vi "Update Digital Acq. Parameters.vi"(8 "error in":errorcluster, 10 "Digital Acquisition Parameters":T1 {"Execution Task Frequency" scale=1.0..100.0}) -> (0 "error out":errorcluster)   [LabVIEW 2020]
doc: "Request to update the Acquisition module with the information required to acquire digital info.\n_____\nCreated using Delacor QMH Event Scripter 6.0.0.121."
uses:
  Shared/DigitalAcquisitionParameters__typedef.ctl
  Shared/Configuration for Acquisitions.lvlib
  Update Digital Acq. Parameters Argument--cluster.ctl
  Acquisition.lvlib
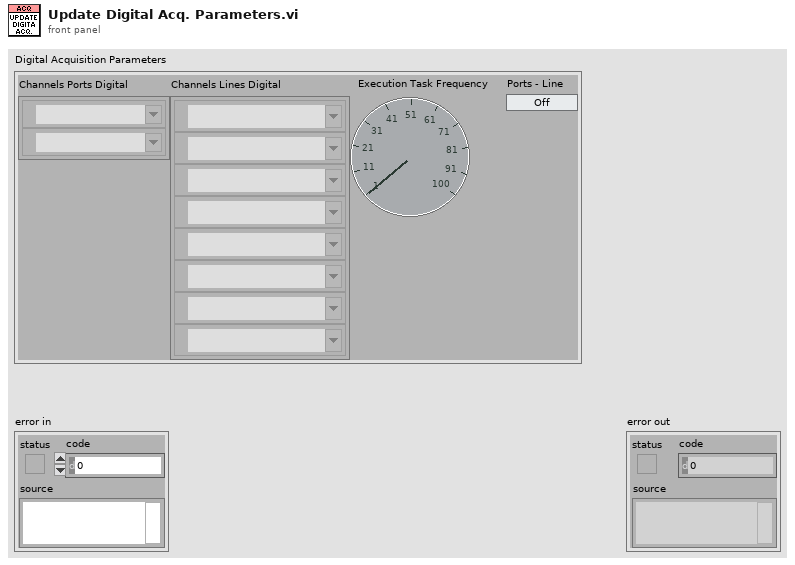
[diagram p1: front panel]
types:
  T1 = typedef "Configuration for Acquisitions.lvlib/DigitalAcquisitionParameters__typedef.ctl" = cluster{"Channels Ports Digital":tag[], "Channels Lines Digital":tag[], "Execution Task Frequency\n":u32, "Ports - Line":bool}
  T2 = typedef "Update Digital Acq. Parameters Argument--cluster.ctl" = cluster{"Digital Acquisition Parameters":T1}
  T3 = typedef "Acquisition.lvlib/Request Events--cluster.ctl" = cluster{"Stop Module":refnum<user-event>, "Show Panel":refnum<user-event>, "Hide Panel":refnum<user-event>, "Get Module Execution Status":refnum<user-event>, "Show Diagram":refnum<user-event>, "Update DAQ Device Name":refnum<user-event>, "Update Total Acquisition Time":refnum<user-event>, "Start Acquisition":refnum<user-event>, "Select Acquisition Type":refnum<user-event>}
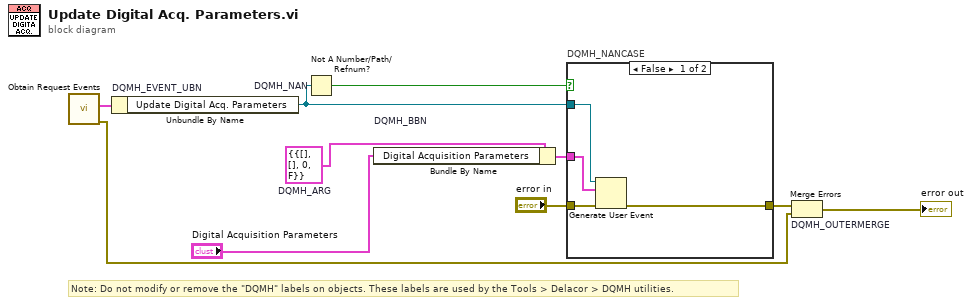
[diagram p0: block diagram]
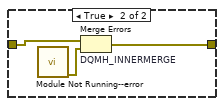
[diagram p2: hidden frame]
diagram:
  w4 = T2 {"Digital Acquisition Parameters"={"Channels Ports Digital"=[], "Channels Lines Digital"=[], "Execution Task Frequency\n"=0, "Ports - Line"=FALSE}}  # DQMH_ARG
  # "Note: Do not modify or remove the \"DQMH\" labels on objects. These labels are used by the Tools > Delacor > DQMH utilities."
  n1 = call "Obtain Request Events.vi"() -> ("error out"=w2:errorcluster, "Acquisition Request Events"=w1:T3)  [unwired: 10 in]
  n2 = Unbundle By Name "DQMH_EVENT_UBN"(w1) -> ("Update Digital Acq. Parameters"=w6:refnum<user-event>)
  n3 = Not A Number/Path/Refnum? "DQMH_NAN"(number/path/refnum=w6) -> (NaN/Path/Refnum?=w7:bool)
  n4 = Bundle By Name "DQMH_BBN"(cluster=w4, "Digital Acquisition Parameters"="Digital Acquisition Parameters") -> (w8:T2)
  n5 = case "DQMH_NANCASE" shown="False" w7 {
    tunnel: "error in" -> [w14 w17]
    tunnel: [w13 w16] -> w5
    tunnel: w6 -> [w12 _]
    tunnel: w8 -> [w11 _]
    frame False {
      n6 = Generate User Event(user event=w12, event data cluster=w11, error in=w14) -> (error out=w13:errorcluster)  [unwired: 1 in, 1 out]
    }
    frame True {
      n7 = call "Module Not Running--error.vi"() -> ("error out"=w15:errorcluster)  [unwired: 11 in]
      n8 = Merge Errors "DQMH_INNERMERGE"(w17, w15) -> (w16:errorcluster)
    }
  }
  n9 = Merge Errors "DQMH_OUTERMERGE"(w5, w2) -> (→"error out":errorcluster)
